vi "ModuleErrEventRefnum.vi"(8 "error in (no error)":errorcluster) -> (0 "error out":errorcluster, 2 "ModuleError Registration Refnum":refnum<event-registration>, 3 "ModuleError":refnum<user-event>)   [LabVIEW 2017, in "Error Handler.lvlib"]
uses:
  Error Handler.lvlib
  Def-ModuleError--Cluster.ctl
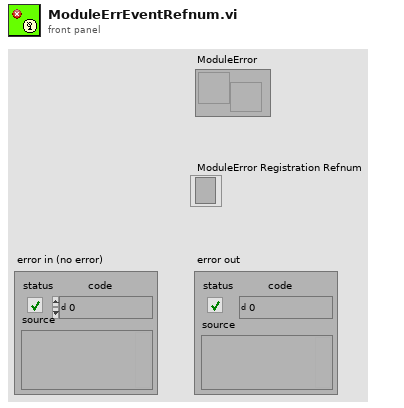
[diagram p1: front panel]
types:
  T1 = typedef "Error Handler.lvlib/Def-ModuleError--Cluster.ctl" = cluster{"Module":string, "error":errorcluster}
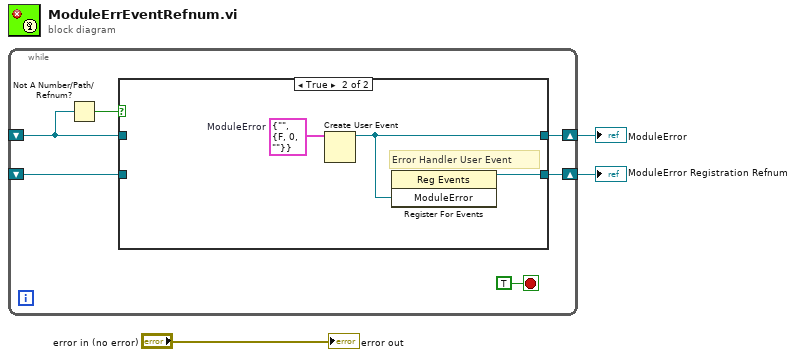
[diagram p0: block diagram]
diagram:
  n1 = while {
    shift-right: [w9] -> w3
    shift-left: _ -> [w6]
    shift-right: [w5] -> w1
    shift-left: _ -> [w4]
    stop <- TRUE stop-if-true
    n2 = Not A Number/Path/Refnum?(number/path/refnum=w6) -> (NaN/Path/Refnum?=w7:bool)
    n3 = case shown="True" w7 {
      tunnel: [w11 w13] -> w9
      tunnel: w6 -> [w11 _]
      tunnel: [w10 w12] -> w5
      tunnel: w4 -> [w10 _]
      frame False {
      }
      frame True {
        w14 = T1 {"Module"="", "error"={"status"=FALSE, "code"=0, "source"=""}}  # ModuleError
        # "Error Handler User Event"
        n4 = Create User Event(user event datatype=w14) -> (user event=w13:refnum<user-event>)  [unwired: 1 in, 1 out]
        n5 = register-events(w13) -> (reference out=w12:refnum<event-registration>)  [unwired: 2 in, 1 out]
      }
    }
  }
  "ModuleError" <- w3
  "ModuleError Registration Refnum" <- w1
  "error out" <- "error in (no error)"
